vi "Compare Download Response.vi"(10 "Expected":refnum<class "CANopen Message.lvclass">, 11 "Actual":refnum<class "CANopen Message.lvclass">) -> (3 "Equal?":bool)   [LabVIEW 2024, in "Service Data Object.lvclass"]
uses:
  CANopen Message/CANopen Message.lvclass
  CANopen Message/CANopen Message.lvclass/CANopen Message.ctl
  Service Data Object.lvclass
  Service Data Object.lvclass/Service Data Object.ctl
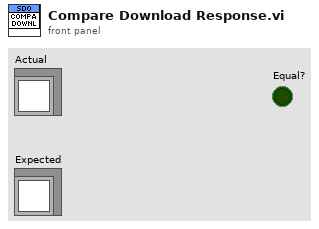
[diagram p1: front panel]
types:
  T1 = typedef "CANopen Master.lvlib/Multiplexor.ctl" = cluster{"Index":u16, "Sub-Index":u8}
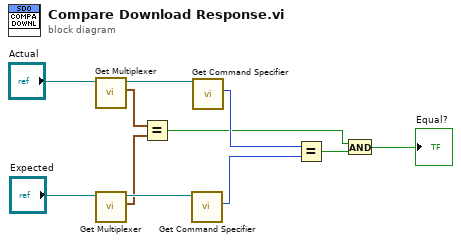
[diagram p0: block diagram]
diagram:
  n1 = call "Get Multiplexer.vi"("CANopen Message in"="Actual") -> ("Multiplexer"=w4:T1, "CANopen Message out"=w6:refnum<class "CANopen Message.lvclass">)  [unwired: 9 in]
  n2 = call "Get Multiplexer.vi"("CANopen Message in"="Expected") -> ("Multiplexer"=w3:T1, "CANopen Message out"=w5:refnum<class "CANopen Message.lvclass">)  [unwired: 9 in]
  n3 = Equal?(x=w4, y=w3) -> (x = y?=w1:bool)
  n4 = call "Get Command Specifier.vi"("CANopen Message in"=w5) -> ("Command Specifier"=w8:u8)  [unwired: 9 in, 1 out]
  n5 = call "Get Command Specifier.vi"("CANopen Message in"=w6) -> ("Command Specifier"=w9:u8)  [unwired: 9 in, 1 out]
  n6 = Equal?(x=w9, y=w8) -> (x = y?=w7:bool)
  n7 = And(x=w1, y=w7) -> (x .and. y?=→"Equal?":bool)
